vi "read_temperature_blueforce.vi"(11 "file (use dialog)":path=path "\\\\192.168.0.4\\log/18-09-20/CH6 T 18-09-20.log") -> (2 "MX Temperature":dbl, 3 "Still Temperature":dbl)   [LabVIEW 2013] (continued)
1.003550E-1\n 20-09-18,17:19:35,1.003100E-1\n 20-09-18,17:19:37,1.008100E-1\n 20-09-18,17:19:40,1.004540E-1\n 20-09-18,17:19:42,1.004540E-1\n 20-09-18,17:19:44,1.011400E-1\n 20-09-18,17:19:46,1.007830E-1\n 20-09-18,17:19:49,1.006880E-1\n 20-09-18,17:19:51,1.005400E-1\n 20-09-18,17:19:53,1.002950E-1\n 20-09-18,17:19:55,1.003440E-1\n 20-09-18,17:19:58,1.003440E-1\n 20-09-18,17:20:00,1.011370E-1\n 20-09-18,17:20:02,1.008280E-1\n 20-09-18,17:20:04,1.006410E-1\n 20-09-18,17:20:07,9.978940E-2\n 20-09-18,17:20:09,9.944410E-2\n 20-09-18,17:20:11,9.896930E-2\n 20-09-18,17:20:13,9.896930E-2\n 20-09-18,17:20:16,9.619440E-2\n 20-09-18,17:20:18,9.739140E-2\n 20-09-18,17:20:20,9.786550E-2\n 20-09-18,17:20:22,9.802170E-2\n 20-09-18,17:20:25,9.851810E-2\n 20-09-18,17:20:27,9.879560E-2\n 20-09-18,17:20:29,9.879560E-2\n 20-09-18,17:20:31,1.018210E-1\n 20-09-18,17:20:34,1.008780E-1\n 20-09-18,17:20:36,1.003490E-1\n 20-09-18,17:20:38,1.002940E-1\n 20-09-18,17:20:40,1.003760E-1\n 20-09-18,17:20:43,1.006140E-1\n 20-09-18,17:20:45,1.006420E-1\n 20-09-18,17:20:47,1.007820E-1\n 20-09-18,17:20:49,9.991960E-2\n 20-09-18,17:20:52,1.001710E-1\n 20-09-18,17:20:54,1.001460E-1\n 20-09-18,17:20:56,1.000700E-1\n 20-09-18,17:20:58,9.978200E-2\n 20-09-18,17:21:01,9.981910E-2\n 20-09-18,17:21:03,9.723240E-2\n 20-09-18,17:21:05,9.977960E-2\n 20-09-18,17:21:07,1.009220E-1\n 20-09-18,17:21:10,1.013280E-1\n 20-09-18,17:21:12,1.022630E-1\n 20-09-18,17:21:14,1.022890E-1\n 20-09-18,17:21:16,1.022930E-1\n 20-09-18,17:21:19,1.044730E-1\n 20-09-18,17:21:21,1.023510E-1\n 20-09-18,17:21:23,1.018190E-1\n 20-09-18,17:21:25,1.013600E-1\n 20-09-18,17:21:28,1.007900E-1\n 20-09-18,17:21:30,1.001160E-1\n 20-09-18,17:21:32,1.000180E-1\n 20-09-18,17:21:34,1.012400E-1\n 20-09-18,17:21:37,9.946230E-2\n 20-09-18,17:21:39,9.922520E-2\n 20-09-18,17:21:41,9.924580E-2\n 20-09-18,17:21:44,9.924410E-2\n 20-09-18,17:21:46,9.917570E-2\n 20-09-18,17:21:48,9.925390E-2\n 20-09-18,17:21:50,9.608970E-2\n 20-09-18,17:21:52,9.825770E-2\n 20-09-18,17:21:55,9.848700E-2\n 20-09-18,17:21:57,9.844790E-2\n 20-09-18,17:21:59,9.851130E-2\n 20-09-18,17:22:02,9.850660E-2\n 20-09-18,17:22:09,9.816970E-2\n 20-09-18,17:22:10,4.394450E+1\n 20-09-18,17:22:12,1.434560E-1\n 20-09-18,17:22:14,2.382460E-1\n 20-09-18,17:22:16,2.448560E-1\n 20-09-18,17:22:19,2.535750E-1\n 20-09-18,17:22:21,2.665980E-1\n 20-09-18,17:22:23,2.845110E-1\n 20-09-18,17:22:25,2.952960E-1\n 20-09-18,17:22:27,2.952960E-1\n 20-09-18,17:22:30,3.319080E-1\n 20-09-18,17:22:32,3.384030E-1\n 20-09-18,17:22:34,3.423260E-1\n 20-09-18,17:22:36,3.452420E-1\n 20-09-18,17:22:39,3.516330E-1\n 20-09-18,17:22:41,3.561550E-1\n 20-09-18,17:22:43,3.561550E-1\n 20-09-18,17:22:45,3.907060E-1\n 20-09-18,17:22:48,3.900440E-1\n 20-09-18,17:22:50,3.925970E-1\n 20-09-18,17:22:52,3.934750E-1\n 20-09-18,17:22:55,3.999280E-1\n 20-09-18,17:22:57,4.096360E-1\n 20-09-18,17:22:59,4.096360E-1\n 20-09-18,17:23:01,4.345180E-1\n 20-09-18,17:23:04,4.472550E-1\n 20-09-18,17:23:06,4.469450E-1\n 20-09-18,17:23:08,4.550520E-1\n 20-09-18,17:23:10,4.655860E-1\n 20-09-18,17:23:13,4.711370E-1\n 20-09-18,17:23:15,4.711370E-1\n 20-09-18,17:23:17,5.197220E-1\n 20-09-18,17:23:19,5.135270E-1\n 20-09-18,17:23:22,5.132950E-1\n 20-09-18,17:23:24,5.200700E-1\n 20-09-18,17:23:26,5.282430E-1\n 20-09-18,17:23:28,5.404450E-1\n 20-09-18,17:23:31,5.427620E-1\n 20-09-18,17:23:33,6.040430E-1\n 20-09-18,17:23:35,6.015100E-1\n 20-09-18,17:23:37,5.947870E-1\n 20-09-18,17:23:40,6.022180E-1\n 20-09-18,17:23:42,6.064140E-1\n 20-09-18,17:23:44,6.170440E-1\n 20-09-18,17:23:46,6.201170E-1\n 20-09-18,17:23:49,6.463890E-1\n 20-09-18,17:23:51,6.510940E-1\n 20-09-18,17:23:53,6.612340E-1\n 20-09-18,17:23:55,6.706050E-1\n 20-09-18,17:23:57,6.760880E-1\n 20-09-18,17:24:00,6.870680E-1\n 20-09-18,17:24:02,6.925720E-1\n 20-09-18,17:24:04,7.401610E-1\n 20-09-18,17:24:06,7.175350E-1\n 20-09-18,17:24:09,7.307670E-1\n 20-09-18,17:24:11,7.454890E-1\n 20-09-18,17:24:13,7.583790E-1\n 20-09-18,17:24:16,7.694830E-1\n 20-09-18,17:24:18,7.733470E-1\n 20-09-18,17:24:20,8.245770E-1\n 20-09-18,17:24:22,8.306260E-1\n 20-09-18,17:24:29,4.394450E+1\n 20-09-18,17:24:31,8.230880E-1\n 20-09-18,17:24:33,7.905300E-1\n 20-09-18,17:24:36,7.623910E-1\n 20-09-18,17:24:38,7.606500E-1\n 20-09-18,17:24:40,7.511750E-1\n 20-09-18,17:24:42,7.473950E-1\n 20-09-18,17:24:45,7.421170E-1\n 20-09-18,17:24:47,7.421170E-1\n 20-09-18,17:24:49,7.099970E-1\n 20-09-18,17:24:51,7.057380E-1\n 20-09-18,17:24:54,7.007630E-1\n 20-09-18,17:24:56,6.917990E-1\n 20-09-18,17:24:58,6.832040E-1\n 20-09-18,17:25:00,6.809020E-1\n 20-09-18,17:25:03,6.343650E-1\n 20-09-18,17:25:05,6.348470E-1\n 20-09-18,17:25:07,6.343000E-1\n 20-09-18,17:25:09,6.377350E-1\n 20-09-18,17:25:12,6.439630E-1\n 20-09-18,17:25:14,6.401860E-1\n 20-09-18,17:25:16,6.375780E-1\n 20-09-18,17:25:18,6.085490E-1\n 20-09-18,17:25:20,6.024800E-1\n 20-09-18,17:25:23,6.063600E-1\n 20-09-18,17:25:25,6.019000E-1\n 20-09-18,17:25:27,5.985790E-1\n 20-09-18,17:25:30,5.928540E-1\n 20-09-18,17:25:32,5.928540E-1\n 20-09-18,17:25:34,5.930700E-1\n 20-09-18,17:25:36,5.743860E-1\n 20-09-18,17:25:39,5.720530E-1\n 20-09-18,17:25:41,5.709990E-1\n 20-09-18,17:25:43,5.595230E-1\n 20-09-18,17:25:45,5.595100E-1\n 20-09-18,17:25:48,5.595100E-1\n 20-09-18,17:25:50,5.525430E-1\n 20-09-18,17:25:52,5.434470E-1\n 20-09-18,17:25:54,5.332690E-1\n 20-09-18,17:25:57,5.272730E-1\n 20-09-18,17:25:59,5.188400E-1\n 20-09-18,17:26:01,5.184060E-1\n 20-09-18,17:26:03,5.211560E-1\n 20-09-18,17:26:06,5.125710E-1\n 20-09-18,17:26:08,5.169210E-1\n 20-09-18,17:26:10,5.094110E-1\n 20-09-18,17:26:12,5.022340E-1\n 20-09-18,17:26:15,4.936660E-1\n 20-09-18,17:26:17,4.910360E-1\n 20-09-18,17:26:19,4.627970E-1\n 20-09-18,17:26:26,4.832560E-1\n 20-09-18,17:26:27,4.394450E+1\n 20-09-18,17:26:29,4.746970E-1\n 20-09-18,17:26:31,4.594830E-1\n 20-09-18,17:26:34,4.579130E-1\n 20-09-18,17:26:36,4.558290E-1\n 20-09-18,17:26:38,4.488550E-1\n 20-09-18,17:26:40,4.453020E-1\n 20-09-18,17:26:43,4.430280E-1\n 20-09-18,17:26:45,4.454690E-1\n 20-09-18,17:26:47,4.312540E-1\n 20-09-18,17:26:49,4.332730E-1\n 20-09-18,17:26:52,4.336780E-1\n 20-09-18,17:26:54,4.325130E-1\n 20-09-18,17:26:56,4.276130E-1\n 20-09-18,17:26:58,4.263080E-1\n 20-09-18,17:27:01,4.249530E-1\n 20-09-18,17:27:03,4.125900E-1\n 20-09-18,17:27:05,4.129050E-1\n 20-09-18,17:27:07,4.101310E-1\n 20-09-18,17:27:10,4.060110E-1\n 20-09-18,17:27:12,4.028180E-1\n 20-09-18,17:27:14,4.028180E-1\n 20-09-18,17:27:16,3.854790E-1\n 20-09-18,17:27:19,3.825800E-1\n 20-09-18,17:27:21,3.832550E-1\n 20-09-18,17:27:23,3.812040E-1\n 20-09-18,17:27:25,3.815990E-1\n 20-09-18,17:27:28,3.799760E-1\n 20-09-18,17:27:30,3.799760E-1\n 20-09-18,17:27:32,3.778860E-1\n 20-09-18,17:27:34,3.722890E-1\n 20-09-18,17:27:37,3.724340E-1\n 20-09-18,17:27:39,3.674890E-1\n 20-09-18,17:27:41,3.674680E-1\n 20-09-18,17:27:43,3.653540E-1\n 20-09-18,17:27:46,3.653540E-1\n 20-09-18,17:27:48,3.556620E-1\n 20-09-18,17:27:50,3.502610E-1\n 20-09-18,17:27:52,3.515170E-1\n 20-09-18,17:27:55,3.500260E-1\n 20-09-18,17:27:57,3.488960E-1\n 20-09-18,17:27:59,3.482360E-1\n 20-09-18,17:28:01,3.356440E-1\n 20-09-18,17:28:04,3.335550E-1\n 20-09-18,17:28:06,3.390470E-1\n 20-09-18,17:28:08,3.378130E-1\n 20-09-18,17:28:10,3.374060E-1\n 20-09-18,17:28:13,3.343680E-1\n 20-09-18,17:28:15,3.334720E-1\n 20-09-18,17:28:17,3.321790E-1\n 20-09-18,17:28:19,3.282410E-1\n 20-09-18,17:28:22,3.234520E-1\n 20-09-18,17:28:24,3.189060E-1\n 20-09-18,17:28:26,3.165180E-1\n 20-09-18,17:28:28,3.141900E-1\n 20-09-18,17:28:31,3.141900E-1\n 20-09-18,17:28:33,3.038560E-1\n 20-09-18,17:28:35,3.010080E-1\n 20-09-18,17:28:37,3.039260E-1\n 20-09-18,17:28:40,3.024480E-1\n 20-09-18,17:28:42,2.979390E-1\n 20-09-18,17:28:44,2.966510E-1\n 20-09-18,17:28:46,2.966510E-1\n 20-09-18,17:28:49,2.978060E-1\n 20-09-18,17:28:51,2.948630E-1\n 20-09-18,17:28:53,2.901630E-1\n 20-09-18,17:28:55,2.869670E-1\n 20-09-18,17:28:58,2.831210E-1\n 20-09-18,17:29:00,2.818300E-1\n 20-09-18,17:29:02,2.744290E-1\n 20-09-18,17:29:04,2.756930E-1\n 20-09-18,17:29:07,2.746590E-1\n 20-09-18,17:29:09,2.745300E-1\n 20-09-18,17:29:11,2.712410E-1\n 20-09-18,17:29:13,2.701060E-1\n 20-09-18,17:29:16,2.692660E-1\n 20-09-18,17:29:18,2.638190E-1\n 20-09-18,17:29:20,2.613780E-1\n 20-09-18,17:29:22,2.614390E-1\n 20-09-18,17:29:25,2.582390E-1\n 20-09-18,17:29:27,2.573290E-1\n 20-09-18,17:29:29,2.546590E-1\n 20-09-18,17:29:32,2.545410E-1\n 20-09-18,17:29:34,2.518470E-1\n 20-09-18,17:29:36,2.521180E-1\n 20-09-18,17:29:38,2.499520E-1\n 20-09-18,17:29:40,2.480330E-1\n 20-09-18,17:29:43,2.444510E-1\n 20-09-18,17:29:45,2.416540E-1\n 20-09-18,17:29:47,2.416540E-1\n 20-09-18,17:29:49,2.429390E-1\n 20-09-18,17:29:52,2.424050E-1\n 20-09-18,17:29:54,2.393320E-1\n 20-09-18,17:29:56,2.367990E-1\n 20-09-18,17:29:58,2.321840E-1\n 20-09-18,17:30:01,2.298570E-1\n 20-09-18,17:30:03,2.298570E-1\n 20-09-18,17:30:05,2.263710E-1\n 20-09-18,17:30:07,2.257250E-1\n 20-09-18,17:30:10,2.257980E-1\n 20-09-18,17:30:12,2.229320E-1\n 20-09-18,17:30:14,2.208340E-1\n 20-09-18,17:30:16,2.204030E-1\n 20-09-18,17:30:19,2.114880E-1\n 20-09-18,17:30:21,2.158310E-1\n 20-09-18,17:30:23,2.161270E-1\n 20-09-18,17:30:25,2.148520E-1\n 20-09-18,17:30:28,2.130850E-1\n 20-09-18,17:30:30,2.124920E-1\n 20-09-18,17:30:32,2.120450E-1\n 20-09-18,17:30:34,2.104050E-1\n 20-09-18,17:30:37,2.088960E-1\n 20-09-18,17:30:39,2.046760E-1\n 20-09-18,17:30:41,2.041510E-1\n 20-09-18,17:30:43,2.033390E-1\n 20-09-18,17:30:46,2.017570E-1\n 20-09-18,17:30:48,2.017570E-1\n 20-09-18,17:30:50,1.988300E-1\n 20-09-18,17:30:52,1.967390E-1\n 20-09-18,17:30:55,1.964210E-1\n 20-09-18,17:30:57,1.956840E-1\n 20-09-18,17:30:59,1.958610E-1\n 20-09-18,17:31:01,1.950230E-1\n 20-09-18,17:31:04,1.950230E-1\n 20-09-18,17:31:06,1.899010E-1\n 20-09-18,17:31:08,1.878370E-1\n 20-09-18,17:31:10,1.869390E-1\n 20-09-18,17:31:13,1.856220E-1\n 20-09-18,17:31:15,1.841570E-1\n 20-09-18,17:31:17,1.834190E-1\n 20-09-18,17:31:20,1.815290E-1\n 20-09-18,17:31:22,1.817090E-1\n 20-09-18,17:31:24,1.821890E-1\n 20-09-18,17:31:26,1.810650E-1\n 20-09-18,17:31:29,1.792830E-1\n 20-09-18,17:31:31,1.765640E-1\n 20-09-18,17:31:33,1.761130E-1\n 20-09-18,17:31:35,1.779350E-1\n 20-09-18,17:31:38,1.730720E-1\n 20-09-18,17:31:40,1.712790E-1\n 20-09-18,17:31:42,1.709350E-1\n 20-09-18,17:31:44,1.703400E-1\n 20-09-18,17:31:47,1.693050E-1\n 20-09-18,17:31:49,1.693050E-1\n 20-09-18,17:31:51,1.664980E-1\n 20-09-18,17:31:53,1.653560E-1\n 20-09-18,17:31:56,1.641030E-1\n 20-09-18,17:31:58,1.634880E-1\n 20-09-18,17:32:00,1.611330E-1\n 20-09-18,17:32:02,1.606460E-1\n 20-09-18,17:32:05,1.606460E-1\n 20-09-18,17:32:07,1.580510E-1\n 20-09-18,17:32:09,1.588140E-1\n 20-09-18,17:32:11,1.580570E-1\n 20-09-18,17:32:14,1.576590E-1\n 20-09-18,17:32:16,1.559470E-1\n 20-09-18,17:32:18,1.551920E-1\n 20-09-18,17:32:20,1.502620E-1\n 20-09-18,17:32:23,1.493690E-1\n 20-09-18,17:32:25,1.496220E-1\n 20-09-18,17:32:27,1.491650E-1\n 20-09-18,17:32:29,1.487820E-1\n 20-09-18,17:32:32,1.472920E-1\n 20-09-18,17:32:34,1.472570E-1\n 20-09-18,17:32:36,1.446360E-1\n 20-09-18,17:32:38,1.450990E-1\n 20-09-18,17:32:41,1.424930E-1\n 20-09-18,17:32:43,1.426100E-1\n 20-09-18,17:32:45,1.412570E-1\n 20-09-18,17:32:47,1.398590E-1\n 20-09-18,17:32:50,1.400110E-1\n 20-09-18,17:32:52,1.349090E-1\n 20-09-18,17:32:54,1.368070E-1\n 20-09-18,17:32:56,1.375790E-1\n 20-09-18,17:32:59,1.375740E-1\n 20-09-18,17:33:01,1.384090E-1\n 20-09-18,17:33:03,1.383900E-1\n 20-09-18,17:33:06,1.386750E-1\n 20-09-18,17:33:08,1.362520E-1\n 20-09-18,17:33:10,1.389960E-1\n 20-09-18,17:33:12,1.389790E-1\n 20-09-18,17:33:15,1.389920E-1\n 20-09-18,17:33:17,1.391900E-1\n 20-09-18,17:33:19,1.394480E-1\n 20-09-18,17:33:21,1.397630E-1\n 20-09-18,17:33:24,1.442280E-1\n 20-09-18,17:33:26,1.425060E-1\n 20-09-18,17:33:28,1.422990E-1\n 20-09-18,17:33:30,1.413730E-1\n 20-09-18,17:33:33,1.408800E-1\n 20-09-18,17:33:35,1.400570E-1\n 20-09-18,17:33:37,1.399870E-1\n 20-09-18,17:33:39,1.393690E-1\n 20-09-18,17:33:42,1.400400E-1\n 20-09-18,17:33:44,1.409940E-1\n 20-09-18,17:33:46,1.404900E-1\n 20-09-18,17:33:48,1.412640E-1\n 20-09-18,17:33:51,1.397430E-1\n 20-09-18,17:33:53,1.394380E-1\n 20-09-18,17:33:55,1.354590E-1\n 20-09-18,17:33:57,1.370790E-1\n 20-09-18,17:34:00,1.387140E-1\n 20-09-18,17:34:02,1.394170E-1\n 20-09-18,17:34:04,1.400810E-1\n 20-09-18,17:34:06,1.401880E-1\n 20-09-18,17:34:08,1.404650E-1\n 20-09-18,17:34:11,1.404650E-1\n 20-09-18,17:34:13,1.416280E-1\n 20-09-18,17:34:15,1.421550E-1\n 20-09-18,17:34:18,1.424520E-1\n 20-09-18,17:34:20,1.424870E-1\n 20-09-18,17:34:22,1.421430E-1\n 20-09-18,17:34:24,1.415370E-1\n 20-09-18,17:34:27,1.415370E-1\n 20-09-18,17:34:29,1.395640E-1\n 20-09-18,17:34:31,1.395150E-1\n 20-09-18,17:34:33,1.397920E-1\n 20-09-18,17:34:36,1.395380E-1\n 20-09-18,17:34:38,1.392860E-1\n 20-09-18,17:34:40,1.392380E-1\n 20-09-18,17:34:42,1.392380E-1\n 20-09-18,17:34:45,1.366050E-1\n 20-09-18,17:34:47,1.372790E-1\n 20-09-18,17:34:49,1.379720E-1\n 20-09-18,17:34:51,1.386800E-1\n 20-09-18,17:34:54,1.393580E-1\n 20-09-18,17:34:56,1.406050E-1\n 20-09-18,17:34:58,1.406050E-1\n 20-09-18,17:35:00,1.444190E-1\n 20-09-18,17:35:03,1.426350E-1\n 20-09-18,17:35:05,1.422680E-1\n 20-09-18,17:35:07,1.424110E-1\n 20-09-18,17:35:09,1.421470E-1\n 20-09-18,17:35:12,1.417140E-1\n 20-09-18,17:35:14,1.417140E-1\n 20-09-18,17:35:16,1.385560E-1\n 20-09-18,17:35:18,1.398480E-1\n 20-09-18,17:35:21,1.402220E-1\n 20-09-18,17:35:23,1.402070E-1\n 20-09-18,17:35:25,1.400320E-1\n 20-09-18,17:35:28,1.399420E-1\n 20-09-18,17:35:30,1.399420E-1\n 20-09-18,17:35:32,1.413960E-1\n 20-09-18,17:35:34,1.418340E-1\n 20-09-18,17:35:37,1.419030E-1\n 20-09-18,17:35:39,1.415460E-1\n 20-09-18,17:35:41,1.411720E-1\n 20-09-18,17:35:43,1.417440E-1\n 20-09-18,17:35:46,1.415180E-1\n 20-09-18,17:35:48,1.406040E-1\n 20-09-18,17:35:50,1.410110E-1\n 20-09-18,17:35:52,1.401270E-1\n 20-09-18,17:35:55,1.396100E-1\n 20-09-18,17:35:57,1.392750E-1\n 20-09-18,17:35:59,1.390290E-1\n 20-09-18,17:36:01,1.390990E-1\n 20-09-18,17:36:04,1.413980E-1\n 20-09-18,17:36:06,1.416770E-1\n 20-09-18,17:36:08,1.408510E-1\n 20-09-18,17:36:10,1.402020E-1\n 20-09-18,17:36:13,1.397680E-1\n 20-09-18,17:36:15,1.391470E-1\n 20-09-18,17:36:17,1.387820E-1\n 20-09-18,17:36:19,1.394540E-1\n 20-09-18,17:36:22,1.406640E-1\n 20-09-18,17:36:24,1.401830E-1\n 20-09-18,17:36:26,1.402610E-1\n 20-09-18,17:36:29,1.398400E-1\n 20-09-18,17:36:31,1.400440E-1\n 20-09-18,17:36:33,1.399740E-1\n 20-09-18,17:36:35,1.427320E-1\n 20-09-18,17:36:38,1.425060E-1\n 20-09-18,17:36:40,1.419520E-1\n 20-09-18,17:36:42,1.416970E-1\n 20-09-18,17:36:44,1.418840E-1\n 20-09-18,17:36:47,1.416080E-1\n 20-09-18,17:36:49,1.415500E-1\n 20-09-18,17:36:51,1.415500E-1\n 20-09-18,17:36:53,1.428920E-1\n 20-09-18,17:36:55,1.417430E-1\n 20-09-18,17:36:58,1.419190E-1\n 20-09-18,17:37:00,1.418720E-1\n 20-09-18,17:37:02,1.405670E-1\n 20-09-18,17:37:04,1.396160E-1\n 20-09-18,17:37:07,1.396160E-1\n 20-09-18,17:37:09,1.378870E-1\n 20-09-18,17:37:11,1.362750E-1\n 20-09-18,17:37:14,1.360980E-1\n 20-09-18,17:37:16,1.354440E-1\n 20-09-18,17:37:18,1.349580E-1\n 20-09-18,17:37:20,1.353770E-1\n 20-09-18,17:37:23,1.353770E-1\n 20-09-18,17:37:25,1.369060E-1\n 20-09-18,17:37:27,1.363170E-1\n 20-09-18,17:37:29,1.369030E-1\n 20-09-18,17:37:32,1.376340E-1\n 20-09-18,17:37:34,1.376640E-1\n 20-09-18,17:37:36,1.383100E-1\n 20-09-18,17:37:38,1.383100E-1\n 20-09-18,17:37:41,1.382150E-1\n 20-09-18,17:37:43,1.395820E-1\n 20-09-18,17:37:45,1.415260E-1\n 20-09-18,17:37:47,1.421520E-1\n 20-09-18,17:37:50,1.441930E-1\n 20-09-18,17:37:52,1.438390E-1\n 20-09-18,17:37:54,1.438390E-1\n 20-09-18,17:37:57,1.474730E-1\n 20-09-18,17:37:59,1.451390E-1\n 20-09-18,17:38:01,1.447460E-1\n 20-09-18,17:38:03,1.441570E-1\n 20-09-18,17:38:05,1.432240E-1\n 20-09-18,17:38:08,1.428590E-1\n 20-09-18,17:38:10,1.428590E-1\n 20-09-18,17:38:12,1.447180E-1\n 20-09-18,17:38:14,1.412430E-1\n 20-09-18,17:38:17,1.415420E-1\n 20-09-18,17:38:19,1.410000E-1\n 20-09-18,17:38:21,1.401190E-1\n 20-09-18,17:38:23,1.397290E-1\n 20-09-18,17:38:26,1.394970E-1\n 20-09-18,17:38:28,1.394520E-1\n 20-09-18,17:38:30,1.398520E-1\n 20-09-18,17:38:32,1.396600E-1\n 20-09-18,17:38:35,1.397530E-1\n 20-09-18,17:38:37,1.398000E-1\n 20-09-18,17:38:39,1.406850E-1\n 20-09-18,17:38:41,1.407400E-1\n 20-09-18,17:38:44,1.400250E-1\n 20-09-18,17:38:46,1.407660E-1\n 20-09-18,17:38:48,1.400360E-1\n 20-09-18,17:38:51,1.404940E-1\n 20-09-18,17:38:53,1.403650E-1\n 20-09-18,17:38:55,1.403170E-1\n 20-09-18,17:38:57,1.401360E-1\n 20-09-18,17:39:00,1.354910E-1\n 20-09-18,17:39:02,1.376820E-1\n 20-09-18,17:39:04,1.393490E-1\n 20-09-18,17:39:06,1.394160E-1\n 20-09-18,17:39:08,1.398000E-1\n 20-09-18,17:39:11,1.401630E-1\n 20-09-18,17:39:13,1.398260E-1\n 20-09-18,17:39:15,1.367300E-1\n 20-09-18,17:39:17,1.385670E-1\n 20-09-18,17:39:20,1.391440E-1\n 20-09-18,17:39:22,1.395240E-1\n 20-09-18,17:39:24,1.397540E-1\n 20-09-18,17:39:26,1.386530E-1\n 20-09-18,17:39:29,1.384110E-1\n 20-09-18,17:39:31,1.384110E-1\n 20-09-18,17:39:33,1.368100E-1\n 20-09-18,17:39:35,1.361160E-1\n 20-09-18,17:39:38,1.365050E-1\n 20-09-18,17:39:40,1.368130E-1\n 20-09-18,17:39:42,1.371940E-1\n 20-09-18,17:39:44,1.377100E-1\n 20-09-18,17:39:47,1.377100E-1\n 20-09-18,17:39:49,1.391140E-1\n 20-09-18,17:39:51,1.394180E-1\n 20-09-18,17:39:53,1.397220E-1\n 20-09-18,17:39:56,1.395860E-1\n 20-09-18,17:39:58,1.400010E-1\n 20-09-18,17:40:00,1.402070E-1\n 20-09-18,17:40:02,1.402070E-1\n 20-09-18,17:40:05,1.405000E-1\n 20-09-18,17:40:07,1.399660E-1\n 20-09-18,17:40:09,1.401720E-1\n 20-09-18,17:40:11,1.400960E-1\n 20-09-18,17:40:14,1.401690E-1\n 20-09-18,17:40:16,1.401950E-1\n 20-09-18,17:40:18,1.401950E-1\n 20-09-18,17:40:21,1.435400E-1\n 20-09-18,17:40:23,1.421750E-1\n 20-09-18,17:40:25,1.414780E-1\n 20-09-18,17:40:27,1.412580E-1\n 20-09-18,17:40:30,1.406550E-1\n 20-09-18,17:40:32,1.402260E-1\n 20-09-18,17:40:34,1.402220E-1\n 20-09-18,17:40:36,1.364060E-1\n 20-09-18,17:40:38,1.400550E-1\n 20-09-18,17:40:41,1.402340E-1\n 20-09-18,17:40:43,1.399550E-1\n 20-09-18,17:40:45,1.402430E-1\n 20-09-18,17:40:47,1.398270E-1\n 20-09-18,17:40:50,1.399890E-1\n 20-09-18,17:40:52,1.422010E-1\n 20-09-18,17:40:54,1.414120E-1\n 20-09-18,17:40:57,1.406060E-1\n 20-09-18,17:40:59,1.399070E-1\n 20-09-18,17:41:01,1.392040E-1\n 20-09-18,17:41:03,1.388570E-1\n 20-09-18,17:41:05,1.387010E-1\n 20-09-18,17:41:08,1.393070E-1\n 20-09-18,17:41:10,1.398410E-1\n 20-09-18,17:41:12,1.398700E-1\n 20-09-18,17:41:14,1.402720E-1\n 20-09-18,17:41:17,1.404960E-1\n 20-09-18,17:41:19,1.407630E-1\n 20-09-18,17:41:21,1.410330E-1\n 20-09-18,17:41:23,1.375250E-1\n 20-09-18,17:41:26,1.392560E-1\n 20-09-18,17:41:28,1.393890E-1\n 20-09-18,17:41:30,1.390170E-1\n 20-09-18,17:41:33,1.388100E-1\n 20-09-18,17:41:35,1.393250E-1\n 20-09-18,17:41:37,1.394970E-1\n 20-09-18,17:41:39,1.409600E-1\n 20-09-18,17:41:42,1.414100E-1\n 20-09-18,17:41:44,1.422700E-1\n 20-09-18,17:41:46,1.422060E-1\n 20-09-18,17:41:48,1.418720E-1\n 20-09-18,17:41:51,1.412150E-1\n 20-09-18,17:41:53,1.413060E-1\n 20-09-18,17:41:55,1.413060E-1\n 20-09-18,17:41:57,1.391900E-1\n 20-09-18,17:42:00,1.392580E-1\n 20-09-18,17:42:02,1.393210E-1\n 20-09-18,17:42:04,1.394050E-1\n 20-09-18,17:42:06,1.386440E-1\n 20-09-18,17:42:09,1.393240E-1\n 20-09-18,17:42:11,1.393240E-1\n 20-09-18,17:42:13,1.385650E-1\n 20-09-18,17:42:15,1.396120E-1\n 20-09-18,17:42:18,1.392510E-1\n 20-09-18,17:42:20,1.396930E-1\n 20-09-18,17:42:22,1.390150E-1\n 20-09-18,17:42:24,1.386920E-1\n 20-09-18,17:42:27,1.386920E-1\n 20-09-18,17:42:29,1.421350E-1\n 20-09-18,17:42:31,1.420160E-1\n 20-09-18,17:42:34,1.407540E-1\n 20-09-18,17:42:36,1.406610E-1\n 20-09-18,17:42:38,1.405470E-1\n 20-09-18,17:42:40,1.404330E-1\n 20-09-18,17:42:43,1.404330E-1\n 20-09-18,17:42:45,1.428940E-1\n 20-09-18,17:42:47,1.410720E-1\n 20-09-18,17:42:49,1.411940E-1\n 20-09-18,17:42:52,1.405620E-1\n 20-09-18,17:42:54,1.401880E-1\n 20-09-18,17:42:56,1.402050E-1\n 20-09-18,17:42:58,1.402050E-1\n 20-09-18,17:43:01,1.396290E-1\n 20-09-18,17:43:03,1.386020E-1\n 20-09-18,17:43:05,1.387990E-1\n 20-09-18,17:43:07,1.384980E-1\n 20-09-18,17:43:10,1.385080E-1\n 20-09-18,17:43:12,1.384650E-1\n 20-09-18,17:43:14,1.384650E-1\n 20-09-18,17:43:16,1.382060E-1\n 20-09-18,17:43:19,1.389990E-1\n 20-09-18,17:43:21,1.397360E-1\n 20-09-18,17:43:23,1.403170E-1\n 20-09-18,17:43:25,1.411810E-1\n 20-09-18,17:43:28,1.419720E-1\n 20-09-18,17:43:30,1.418860E-1\n 20-09-18,17:43:32,1.423960E-1\n 20-09-18,17:43:35,1.407990E-1\n 20-09-18,17:43:37,1.410250E-1\n 20-09-18,17:43:39,1.413570E-1\n 20-09-18,17:43:41,1.414750E-1\n 20-09-18,17:43:44,1.414370E-1\n 20-09-18,17:43:46,1.414570E-1\n 20-09-18,17:43:48,1.440010E-1\n 20-09-18,17:43:50,1.427030E-1\n 20-09-18,17:43:53,1.421630E-1\n 20-09-18,17:43:55,1.423240E-1\n 20-09-18,17:43:57,1.422460E-1\n 20-09-18,17:43:59,1.419100E-1\n 20-09-18,17:44:01,1.418730E-1\n 20-09-18,17:44:04,1.383690E-1\n 20-09-18,17:44:06,1.383030E-1\n 20-09-18,17:44:08,1.386570E-1\n 20-09-18,17:44:10,1.386760E-1\n 20-09-18,17:44:13,1.389390E-1\n 20-09-18,17:44:15,1.398170E-1\n 20-09-18,17:44:17,1.398560E-1\n 20-09-18,17:44:19,1.398560E-1\n 20-09-18,17:44:22,1.387240E-1\n 20-09-18,17:44:24,1.397250E-1\n 20-09-18,17:44:26,1.402850E-1\n 20-09-18,17:44:29,1.402230E-1\n 20-09-18,17:44:31,1.393940E-1\n 20-09-18,17:44:38,4.394450E+1\n 20-09-18,17:44:40,1.357180E-1\n 20-09-18,17:44:42,1.408950E-1\n 20-09-18,17:44:44,1.411780E-1\n 20-09-18,17:44:47,1.412840E-1\n 20-09-18,17:44:49,1.411520E-1\n 20-09-18,17:44:51,1.404030E-1\n 20-09-18,17:44:53,1.394680E-1\n 20-09-18,17:44:56,1.394680E-1\n 20-09-18,17:44:58,1.354750E-1\n 20-09-18,17:45:00,1.362050E-1\n 20-09-18,17:45:03,1.356880E-1\n 20-09-18,17:45:05,1.353320E-1\n 20-09-18,17:45:07,1.345030E-1\n 20-09-18,17:45:09,1.340180E-1\n 20-09-18,17:45:12,1.340180E-1\n 20-09-18,17:45:14,1.388130E-1\n 20-09-18,17:45:16,1.387170E-1\n 20-09-18,17:45:19,1.389230E-1\n 20-09-18,17:45:21,1.386460E-1\n 20-09-18,17:45:23,1.386170E-1\n 20-09-18,17:45:25,1.380890E-1\n 20-09-18,17:45:27,1.380890E-1\n 20-09-18,17:45:30,1.376950E-1\n 20-09-18,17:45:32,1.379110E-1\n 20-09-18,17:45:34,1.376990E-1\n 20-09-18,17:45:36,1.372180E-1\n 20-09-18,17:45:39,1.371350E-1\n 20-09-18,17:45:41,1.372360E-1\n 20-09-18,17:45:43,1.372360E-1\n 20-09-18,17:45:45,1.364030E-1\n 20-09-18,17:45:48,1.352120E-1\n 20-09-18,17:45:50,1.351460E-1\n 20-09-18,17:45:52,1.359730E-1\n 20-09-18,17:45:54,1.366090E-1\n 20-09-18,17:45:57,1.376740E-1\n 20-09-18,17:45:59,1.376740E-1\n 20-09-18,17:46:01,1.356470E-1\n 20-09-18,17:46:04,1.352520E-1\n 20-09-18,17:46:06,1.354380E-1\n 20-09-18,17:46:08,1.356310E-1\n 20-09-18,17:46:10,1.365330E-1\n 20-09-18,17:46:12,1.374000E-1\n 20-09-18,17:46:15,1.374390E-1\n 20-09-18,17:46:17,1.376040E-1\n 20-09-18,17:46:19,1.370570E-1\n 20-09-18,17:46:22,1.371970E-1\n 20-09-18,17:46:24,1.370750E-1\n 20-09-18,17:46:26,1.369670E-1\n 20-09-18,17:46:28,1.371050E-1\n 20-09-18,17:46:31,1.371760E-1\n 20-09-18,17:46:33,1.390100E-1\n 20-09-18,17:46:35,1.383820E-1\n 20-09-18,17:46:37,1.378290E-1\n 20-09-18,17:46:40,1.373050E-1\n 20-09-18,17:46:42,1.370910E-1\n 20-09-18,17:46:44,1.368240E-1\n 20-09-18,17:46:46,1.368370E-1\n 20-09-18,17:46:49,1.382110E-1\n 20-09-18,17:46:51,1.390800E-1\n 20-09-18,17:46:53,1.386970E-1\n 20-09-18,17:46:55,1.387730E-1\n 20-09-18,17:46:58,1.386500E-1\n 20-09-18,17:47:00,1.389100E-1\n 20-09-18,17:47:02,1.386270E-1\n 20-09-18,17:47:04,1.341250E-1\n 20-09-18,17:47:07,1.353580E-1\n 20-09-18,17:47:09,1.362740E-1\n 20-09-18,17:47:11,1.365400E-1\n 20-09-18,17:47:13,1.368920E-1\n 20-09-18,17:47:16,1.362660E-1\n 20-09-18,17:47:18,1.363020E-1\n 20-09-18,17:47:20,1.375790E-1\n 20-09-18,17:47:22,1.381260E-1\n 20-09-18,17:47:25,1.384080E-1\n 20-09-18,17:47:27,1.383430E-1\n 20-09-18,17:47:29,1.374250E-1\n 20-09-18,17:47:31,1.373100E-1\n 20-09-18,17:47:34,1.368450E-1\n 20-09-18,17:47:36,1.410820E-1\n 20-09-18,17:47:38,1.367790E-1\n 20-09-18,17:47:41,1.374770E-1\n 20-09-18,17:47:43,1.374450E-1\n 20-09-18,17:47:45,1.371940E-1\n 20-09-18,17:47:47,1.378300E-1\n 20-09-18,17:47:50,1.373220E-1\n 20-09-18,17:47:52,1.373220E-1\n 20-09-18,17:47:54,1.361340E-1\n 20-09-18,17:47:56,1.354830E-1\n 20-09-18,17:47:59,1.352500E-1\n 20-09-18,17:48:01,1.355640E-1\n 20-09-18,17:48:03,1.358710E-1\n 20-09-18,17:48:05,1.365580E-1\n 20-09-18,17:48:07,1.365580E-1\n 20-09-18,17:48:10,1.389120E-1\n 20-09-18,17:48:12,1.388450E-1\n 20-09-18,17:48:14,1.386250E-1\n 20-09-18,17:48:17,1.378030E-1\n 20-09-18,17:48:19,1.370840E-1\n 20-09-18,17:48:21,1.370500E-1\n 20-09-18,17:48:23,1.370500E-1\n 20-09-18,17:48:26,1.365010E-1\n 20-09-18,17:48:28,1.361240E-1\n 20-09-18,17:48:30,1.361980E-1\n 20-09-18,17:48:32,1.361840E-1\n 20-09-18,17:48:35,1.365450E-1\n 20-09-18,17:48:37,1.371290E-1\n 20-09-18,17:48:39,1.371290E-1\n 20-09-18,17:48:41,1.392890E-1\n 20-09-18,17:48:44,1.397830E-1\n 20-09-18,17:48:46,1.397360E-1\n 20-09-18,17:48:48,1.400920E-1\n 20-09-18,17:48:50,1.405730E-1\n 20-09-18,17:48:53,1.406230E-1\n 20-09-18,17:48:55,1.406230E-1\n 20-09-18,17:48:57,1.355080E-1\n 20-09-18,17:48:59,1.370080E-1\n 20-09-18,17:49:02,1.374290E-1\n 20-09-18,17:49:04,1.375130E-1\n 20-09-18,17:49:06,1.377730E-1\n 20-09-18,17:49:08,1.372290E-1\n 20-09-18,17:49:11,1.372290E-1\n 20-09-18,17:49:13,1.365800E-1\n 20-09-18,17:49:15,1.387150E-1\n 20-09-18,17:49:17,1.387660E-1\n 20-09-18,17:49:20,1.386020E-1\n 20-09-18,17:49:22,1.383050E-1\n 20-09-18,17:49:24,1.379970E-1\n 20-09-18,17:49:26,1.380740E-1\n 20-09-18,17:49:29,1.423730E-1\n 20-09-18,17:49:31,1.403280E-1\n 20-09-18,17:49:33,1.397350E-1\n 20-09-18,17:49:35,1.397020E-1\n 20-09-18,17:49:38,1.396130E-1\n 20-09-18,17:49:40,1.401150E-1\n 20-09-18,17:49:42,1.402830E-1\n 20-09-18,17:49:44,1.392750E-1\n 20-09-18,17:49:47,1.370990E-1\n 20-09-18,17:49:49,1.376610E-1\n 20-09-18,17:49:51,1.383680E-1\n 20-09-18,17:49:53,1.386030E-1\n 20-09-18,17:49:56,1.380120E-1\n 20-09-18,17:49:58,1.378130E-1\n 20-09-18,17:50:00,1.373810E-1\n 20-09-18,17:50:03,1.372940E-1\n 20-09-18,17:50:05,1.371560E-1\n 20-09-18,17:50:07,1.370270E-1\n 20-09-18,17:50:09,1.366520E-1\n 20-09-18,17:50:12,1.362110E-1\n 20-09-18,17:50:14,1.360100E-1\n 20-09-18,17:50:16,1.368020E-1\n 20-09-18,17:50:18,1.345950E-1\n 20-09-18,17:50:21,1.356010E-1\n 20-09-18,17:50:23,1.361590E-1\n 20-09-18,17:50:25,1.365460E-1\n 20-09-18,17:50:27,1.372800E-1\n 20-09-18,17:50:30,1.372270E-1\n 20-09-18,17:50:32,1.358960E-1\n 20-09-18,17:50:34,1.349140E-1\n 20-09-18,17:50:36,1.352700E-1\n 20-09-18,17:50:39,1.356030E-1\n 20-09-18,17:50:41,1.352740E-1\n 20-09-18,17:50:43,1.356210E-1\n 20-09-18,17:50:45,1.356360E-1\n 20-09-18,17:50:48,1.401520E-1\n 20-09-18,17:50:50,1.375760E-1\n 20-09-18,17:50:52,1.378570E-1\n 20-09-18,17:50:54,1.381560E-1\n 20-09-18,17:50:57,1.380110E-1\n 20-09-18,17:50:59,1.380110E-1\n 20-09-18,17:51:01,1.381390E-1\n 20-09-18,17:51:03,1.355010E-1\n 20-09-18,17:51:06,1.363530E-1\n 20-09-18,17:51:08,1.360910E-1\n 20-09-18,17:51:10,1.362330E-1\n 20-09-18,17:51:17,1.366220E-1\n 20-09-18,17:51:19,1.366220E-1\n 20-09-18,17:51:21,1.446570E-1\n 20-09-18,17:51:24,1.410680E-1\n 20-09-18,17:51:26,1.395150E-1\n 20-09-18,17:51:28,1.375210E-1\n 20-09-18,17:51:30,1.366680E-1\n 20-09-18,17:51:33,1.363470E-1\n 20-09-18,17:51:35,1.363470E-1\n 20-09-18,17:51:37,1.352840E-1\n 20-09-18,17:51:39,1.352960E-1\n 20-09-18,17:51:42,1.351980E-1\n 20-09-18,17:51:44,1.349190E-1\n 20-09-18,17:51:46,1.345510E-1\n 20-09-18,17:51:48,1.345300E-1\n 20-09-18,17:51:51,1.345300E-1\n 20-09-18,17:51:53,1.353590E-1\n 20-09-18,17:51:55,1.343050E-1\n 20-09-18,17:51:58,1.342290E-1\n 20-09-18,17:52:00,1.337700E-1\n 20-09-18,17:52:02,1.341100E-1\n 20-09-18,17:52:04,1.345180E-1\n 20-09-18,17:52:07,1.345180E-1\n 20-09-18,17:52:12,4.394450E+1\n 20-09-18,17:52:15,1.348200E-1\n 20-09-18,17:52:17,1.417770E-1\n 20-09-18,17:52:19,1.422170E-1\n 20-09-18,17:52:21,1.427270E-1\n 20-09-18,17:52:24,1.431880E-1\n 20-09-18,17:52:26,1.431690E-1\n 20-09-18,17:52:28,1.430190E-1\n 20-09-18,17:52:30,1.429570E-1\n 20-09-18,17:52:33,1.390120E-1\n 20-09-18,17:52:35,1.401090E-1\n 20-09-18,17:52:37,1.405020E-1\n 20-09-18,17:52:39,1.404400E-1\n 20-09-18,17:52:42,1.406170E-1\n 20-09-18,17:52:44,1.408090E-1\n 20-09-18,17:52:46,1.408610E-1\n 20-09-18,17:52:48,1.388810E-1\n 20-09-18,17:52:50,1.386690E-1\n 20-09-18,17:52:53,1.386210E-1\n 20-09-18,17:52:55,1.390940E-1\n 20-09-18,17:52:57,1.386960E-1\n 20-09-18,17:52:59,1.383400E-1\n 20-09-18,17:53:02,1.384110E-1\n 20-09-18,17:53:04,1.335020E-1\n 20-09-18,17:53:06,1.357240E-1\n 20-09-18,17:53:08,1.366160E-1\n 20-09-18,17:53:11,1.367430E-1\n 20-09-18,17:53:13,1.372710E-1\n 20-09-18,17:53:15,1.376990E-1\n 20-09-18,17:53:17,1.374610E-1\n 20-09-18,17:53:20,1.416330E-1\n 20-09-18,17:53:22,1.404620E-1\n 20-09-18,17:53:24,1.393120E-1\n 20-09-18,17:53:26,1.389570E-1\n 20-09-18,17:53:29,1.388590E-1\n 20-09-18,17:53:31,1.397200E-1\n 20-09-18,17:53:33,1.397780E-1\n 20-09-18,17:53:35,1.397780E-1\n 20-09-18,17:53:38,1.417360E-1\n 20-09-18,17:53:40,1.416460E-1\n 20-09-18,17:53:42,1.413720E-1\n 20-09-18,17:53:44,1.417890E-1\n 20-09-18,17:53:47,1.409040E-1\n 20-09-18,17:53:49,1.409070E-1\n 20-09-18,17:53:51,1.409070E-1\n 20-09-18,17:53:54,1.403420E-1\n 20-09-18,17:53:56,1.403990E-1\n 20-09-18,17:53:58,1.402460E-1\n 20-09-18,17:54:00,1.406000E-1\n 20-09-18,17:54:03,1.409920E-1\n 20-09-18,17:54:05,1.405760E-1\n 20-09-18,17:54:07,1.405760E-1\n 20-09-18,17:54:09,1.389390E-1\n 20-09-18,17:54:12,1.385760E-1\n 20-09-18,17:54:14,1.383650E-1\n 20-09-18,17:54:16,1.384780E-1\n 20-09-18,17:54:18,1.387150E-1\n 20-09-18,17:54:21,1.389760E-1\n 20-09-18,17:54:23,1.389760E-1\n 20-09-18,17:54:25,1.395050E-1\n 20-09-18,17:54:27,1.394360E-1\n 20-09-18,17:54:30,1.395780E-1\n 20-09-18,17:54:32,1.397570E-1\n 20-09-18,17:54:34,1.397640E-1\n 20-09-18,17:54:36,1.403040E-1\n 20-09-18,17:54:39,1.403040E-1\n 20-09-18,17:54:41,1.381870E-1\n 20-09-18,17:54:43,1.386730E-1\n 20-09-18,17:54:45,1.388110E-1\n 20-09-18,17:54:48,1.390460E-1\n 20-09-18,17:54:50,1.395330E-1\n 20-09-18,17:54:52,1.404290E-1\n 20-09-18,17:54:54,1.404290E-1\n 20-09-18,17:54:57,1.424210E-1\n 20-09-18,17:54:59,1.416690E-1\n 20-09-18,17:55:01,1.414180E-1\n 20-09-18,17:55:03,1.413740E-1\n 20-09-18,17:55:06,1.413790E-1\n 20-09-18,17:55:08,1.412790E-1\n 20-09-18,17:55:10,1.415700E-1\n 20-09-18,17:55:13,1.389570E-1\n 20-09-18,17:55:15,1.404370E-1\n 20-09-18,17:55:17,1.410640E-1\n 20-09-18,17:55:19,1.405410E-1\n 20-09-18,17:55:21,1.405430E-1\n 20-09-18,17:55:24,1.394720E-1\n 20-09-18,17:55:26,1.392090E-1\n 20-09-18,17:55:28,1.383930E-1\n 20-09-18,17:55:30,1.392150E-1\n 20-09-18,17:55:33,1.394400E-1\n 20-09-18,17:55:35,1.392930E-1\n 20-09-18,17:55:37,1.392370E-1\n 20-09-18,17:55:39,1.391180E-1\n 20-09-18,17:55:42,1.391360E-1\n 20-09-18,17:55:44,1.364590E-1\n 20-09-18,17:55:46,1.387810E-1\n 20-09-18,17:55:48,1.393550E-1\n 20-09-18,17:55:55,1.395780E-1\n 20-09-18,17:55:57,1.395780E-1\n 20-09-18,17:55:59,1.449480E-1\n 20-09-18,17:56:01,1.411930E-1\n 20-09-18,17:56:04,1.415140E-1\n 20-09-18,17:56:06,1.412930E-1\n 20-09-18,17:56:08,1.397510E-1\n 20-09-18,17:56:10,1.387180E-1\n 20-09-18,17:56:13,1.384260E-1\n 20-09-18,17:56:15,1.376540E-1\n 20-09-18,17:56:17,1.347810E-1\n 20-09-18,17:56:19,1.345600E-1\n 20-09-18,17:56:22,1.344030E-1\n 20-09-18,17:56:24,1.338770E-1\n 20-09-18,17:56:26,1.333980E-1\n 20-09-18,17:56:28,1.331970E-1\n 20-09-18,17:56:31,1.342520E-1\n 20-09-18,17:56:33,1.344600E-1\n 20-09-18,17:56:35,1.346330E-1\n 20-09-18,17:56:37,1.343260E-1\n 20-09-18,17:56:40,1.344150E-1\n 20-09-18,17:56:42,1.342850E-1\n 20-09-18,17:56:44,1.343140E-1\n 20-09-18,17:56:47,1.338040E-1\n 20-09-18,17:56:49,1.340700E-1\n 20-09-18,17:56:51,1.338120E-1\n 20-09-18,17:56:53,1.340780E-1\n 20-09-18,17:56:56,1.344730E-1\n 20-09-18,17:56:58,1.347540E-1\n 20-09-18,17:57:00,1.350130E-1\n 20-09-18,17:57:02,1.313970E-1\n 20-09-18,17:57:05,1.342640E-1\n 20-09-18,17:57:07,1.345660E-1\n 20-09-18,17:57:09,1.344980E-1\n 20-09-18,17:57:11,1.338950E-1\n 20-09-18,17:57:14,1.332900E-1\n 20-09-18,17:57:16,1.329330E-1\n 20-09-18,17:57:18,1.317930E-1\n 20-09-18,17:57:20,1.314640E-1\n 20-09-18,17:57:23,1.322000E-1\n 20-09-18,17:57:25,1.320160E-1\n 20-09-18,17:57:27,1.324460E-1\n 20-09-18,17:57:29,1.324960E-1\n 20-09-18,17:57:32,1.322710E-1\n 20-09-18,17:57:34,1.362880E-1\n 20-09-18,17:57:36,1.339980E-1\n 20-09-18,17:57:38,1.340860E-1\n 20-09-18,17:57:41,1.339470E-1\n 20-09-18,17:57:43,1.336460E-1\n 20-09-18,17:57:45,1.338340E-1\n 20-09-18,17:57:47,1.336220E-1\n 20-09-18,17:57:50,1.336220E-1\n 20-09-18,17:57:52,1.352730E-1\n 20-09-18,17:57:54,1.364120E-1\n 20-09-18,17:57:56,1.359660E-1\n 20-09-18,17:57:59,1.360180E-1\n 20-09-18,17:58:01,1.362610E-1\n 20-09-18,17:58:03,1.365180E-1\n 20-09-18,17:58:05,1.365180E-1\n 20-09-18,17:58:08,1.366610E-1\n 20-09-18,17:58:10,1.366470E-1\n 20-09-18,17:58:12,1.375080E-1\n 20-09-18,17:58:14,1.377450E-1\n 20-09-18,17:58:22,1.397310E-1\n 20-09-18,17:58:22,1.397310E-1\n 20-09-18,17:58:24,1.397310E-1\n 20-09-18,17:58:27,1.457780E-1\n 20-09-18,17:58:29,1.441980E-1\n 20-09-18,17:58:31,1.436410E-1\n 20-09-18,17:58:33,1.423810E-1\n 20-09-18,17:58:36,1.420130E-1\n 20-09-18,17:58:38,1.416860E-1\n"
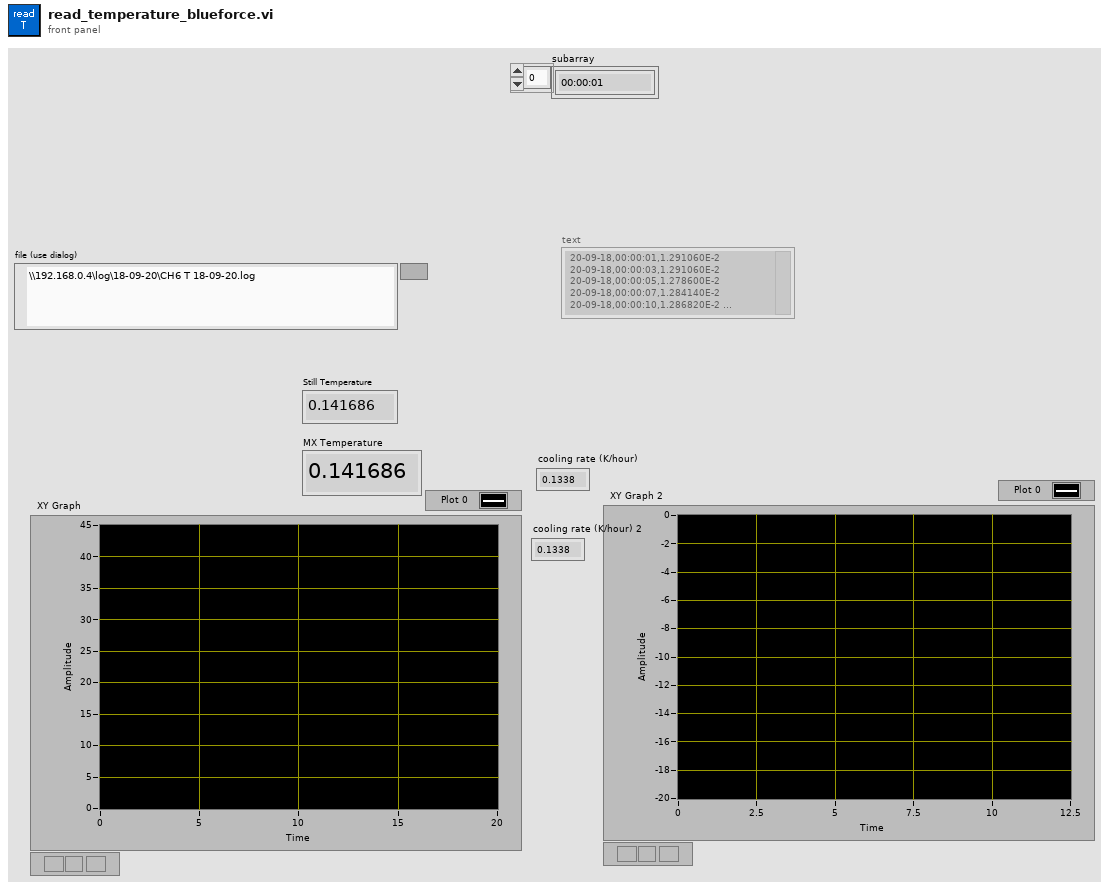
[diagram p1: front panel]
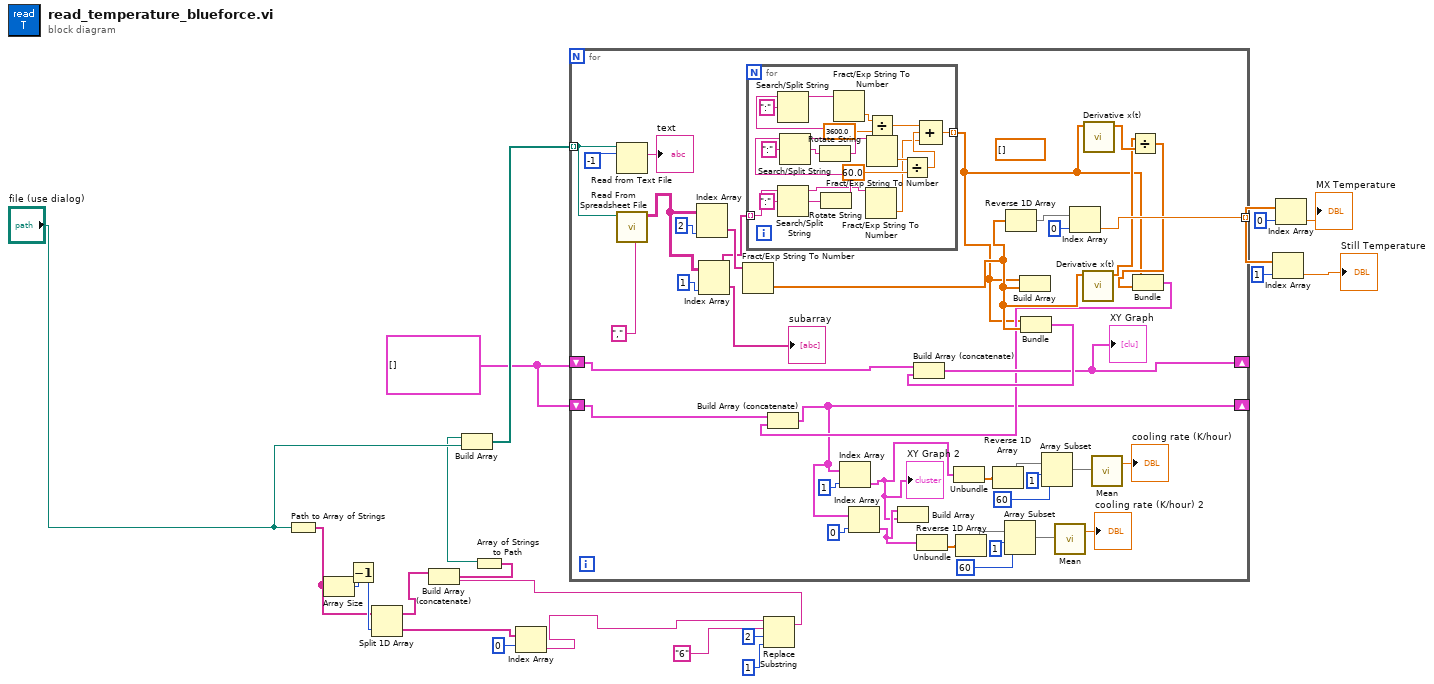
[diagram p0: block diagram]
diagram:
  w1 = cluster{dbl[], dbl[]}[] []
  n1 = Path to Array of Strings(0:"file (use dialog)") -> (2:w13:string[])  [unwired: 1 out]
  n2 = Array Size(array=w13) -> (size(s)=w21:i32)
  n3 = Decrement(x=w21) -> (x-1=w14:i32)
  n4 = Split 1D Array(array=w13, index=w14) -> (first subarray=w12:string[], second subarray=w20:string[])
  n5 = Index Array(array=w20, index=0) -> (element=w18:string)
  n6 = Replace Substring(2:1 ("offset (0)"), 3:2 ("offset (0)"), 4:"6", 5:w18) -> (1:w11:string)  [unwired: 1 out]
  n7 = Build Array (concatenate)(w12, w11) -> (w10:string[])
  n8 = Array of Strings to Path(0:w10) -> (2:w8:path)  [unwired: 1 in]
  n9 = Build Array(w8, "file (use dialog)") -> (w7:path[])
  n10 = for {
    tunnel: w7 -> [w52] mode=indexing
    tunnel: [w51] -> w6 mode=indexing
    shift-right: [w46] -> _
    shift-left: w1 -> [w48]
    shift-right: [w30] -> _
    shift-left: w1 -> [w44]
    (unwired) ext[] []
    n11 = Read from Text File(file (use dialog)=w52, count=-1) -> (text=→"text":string)  [unwired: 2 in, 3 out]
    n12 = call-poly <vilib>:"Read From Spreadsheet File.vi"("delimiter (\\t)"="," ("delimiter (\\t)"), "file path (dialog if empty)"=w52) -> ("all rows"=w53:string[][])  [unwired: 5 in, 4 out]
    n13 = Index Array(array=w53, index (col)=2 ("index (row)")) -> (element=w50:string[])  [unwired: 1 in]
    n14 = Index Array(array=w53, index (col)=1 ("index (row)")) -> (element=w49:string[])  [unwired: 1 in]
    "subarray" <- w49
    n15 = Fract/Exp String To Number(string=w50) -> (number=w45:dbl[])  [unwired: 3 in, 1 out]
    n16 = for {
      tunnel: w49 -> [w79] mode=indexing
      tunnel: [w61] -> w39 mode=indexing
      n17 = Search/Split String(string=w79, search string/char (-)=":") -> (substring before match=w71:string, match + rest of string=w76:string)  [unwired: 1 in, 1 out]
      n18 = Rotate String(1:w76) -> (0:w75:string)
      n19 = Search/Split String(string=w75, search string/char (-)=":") -> (substring before match=w70:string, match + rest of string=w74:string)  [unwired: 1 in, 1 out]
      n20 = Rotate String(1:w74) -> (0:w72:string)
      n21 = Search/Split String(string=w72, search string/char (-)=":") -> (substring before match=w69:string)  [unwired: 1 in, 2 out]
      n22 = Fract/Exp String To Number(string=w69) -> (number=w66:dbl)  [unwired: 3 in, 1 out]
      n23 = Fract/Exp String To Number(string=w71) -> (number=w62:dbl)  [unwired: 3 in, 1 out]
      n24 = Divide(x=w66, y=3600.0) -> (x/y=w64:dbl)
      n25 = Fract/Exp String To Number(string=w70) -> (number=w68:dbl)  [unwired: 3 in, 1 out]
      n26 = Divide(x=w68, y=60.0) -> (x/y=w63:dbl)
      n27 = Compound Arithmetic op=ADD(w64, w63, w62) -> (w61:dbl)
    }
    n28 = Reverse 1D Array(array=w45) -> (reversed array=w56:dbl[])
    n29 = Build Array(w39, w45) -> ()  [unwired: 1 out]
    n30 = Bundle(w39, w45) -> (w47:cluster{dbl[], dbl[]})  [unwired: 1 in]
    n31 = Build Array (concatenate)(w48, w47) -> (w46:cluster{dbl[], dbl[]}[])
    "XY Graph" <- w46
    n32 = Index Array(array=w56, index=0) -> (element=w51:dbl)
    n33 = call <vilib>:"Derivative x(t).vi"("X"=w45) -> ("dX/dt"=w41:dbl[])  [unwired: 9 in, 1 out]
    n34 = call <vilib>:"Derivative x(t).vi"("X"=w39) -> ("dX/dt"=w42:dbl[])  [unwired: 9 in, 1 out]
    n35 = Divide(x=w41, y=w42) -> (x/y=w40:dbl[])
    n36 = Bundle(w39, w40) -> (w43:cluster{dbl[], dbl[]})  [unwired: 1 in]
    n37 = Build Array (concatenate)(w44, w43) -> (w30:cluster{dbl[], dbl[]}[])
    n38 = Index Array(array=w30, index=1) -> (element=w22:cluster{dbl[], dbl[]})
    "XY Graph 2" <- w22
    n39 = Index Array(array=w30, index=0) -> (element=w23:cluster{dbl[], dbl[]})
    n40 = Build Array(w23, w22) -> ()  [unwired: 1 out]
    n41 = Unbundle(w23) -> (w29:dbl[])  [unwired: 1 out]
    n42 = Unbundle(w22) -> (w37:dbl[])  [unwired: 1 out]
    n43 = Reverse 1D Array(array=w29) -> (reversed array=w28:dbl[])
    n44 = Reverse 1D Array(array=w37) -> (reversed array=w36:dbl[])
    n45 = Array Subset(array=w28, index=1, length=60) -> (w25:dbl[])
    n46 = Array Subset(array=w36, index=1, length=60) -> (w33:dbl[])
    n47 = call-poly <vilib>:"Mean.vi"("X"=w25) -> ("mean"=→"cooling rate (K/hour) 2":dbl)  [unwired: 1 out]
    n48 = call-poly <vilib>:"Mean.vi"("X"=w33) -> ("mean"=→"cooling rate (K/hour)":dbl)  [unwired: 1 out]
  }
  n49 = Index Array(array=w6, index=1) -> (element=→"Still Temperature":dbl)
  n50 = Index Array(array=w6, index=0) -> (element=→"MX Temperature":dbl)
